vi "read file.vi"(10 "file name":string, 11 "file path (dialog if empty)":path) -> (2 "2d data":dbl[][](array[numeric]), 3 "1d Data":dbl[](array[numeric]))   [LabVIEW 2024]
uses:
  <vilib>/Utility/file.llb/Read Delimited Spreadsheet (DBL).vi
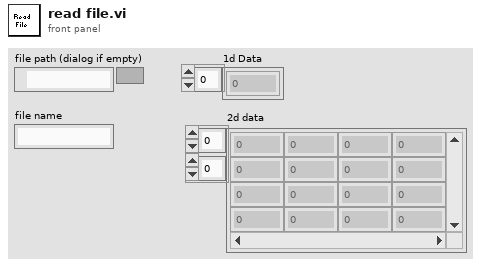
[diagram p1: front panel]
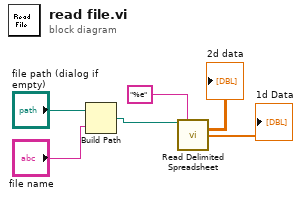
[diagram p0: block diagram]
diagram:
  n1 = Build Path(base path="file path (dialog if empty)", name or relative path="file name") -> (appended path=w4:path)
  n2 = call-poly <vilib>:"Read Delimited Spreadsheet.vi"("file path (dialog if empty)"=w4, "format (%.3f)"="%e") -> ("all rows"=→"2d data":dbl[][], "first row"=→"1d Data":dbl[])  [unwired: 8 in, 4 out]
